vi "initializeGlobals.vi"   [LabVIEW 2015]
uses:
  X:/Lab/Labmembers/Shane Nichols/Labview/InstrumentControl20190423/general_utilities.llb/multiDeviceSynchronization.ctl
  X:/Lab/Labmembers/Shane Nichols/Labview/InstrumentControl20190423/general_utilities.llb/GlobalRefs.vi
  <vilib>/AdaptiveUpright/globalRefs_rigDependent.vi
types:
  T1 = cluster{"galvoX":cluster{"name":string, "physicalChannel":tag}, "galvoY":cluster{"name":string, "physicalChannel":tag}, "mod488":cluster{"name":string, "physicalChannel":tag}, "modTiSaph":cluster{"name":string, "physicalChannel":tag}, "shutter488":cluster{"name":string, "physicalChannel":tag}, "shutterTiSaph":cluster{"name":string, "physicalChannel":tag}, " shutter635":cluster{"name":string, "physicalChannel":tag}, " shutter635-2":cluster{"name":string, "physicalChannel":tag}, "triggerCamera":cluster{"name":string, "physicalChannel":tag}, "triggerBlackfly":cluster{"name":string, "physicalChannel":tag}}
  T2 = cluster{"PMTA":cluster{"name":string, "physicalChannel":tag, "Active?":bool}, "PMTB":cluster{"name":string, "physicalChannel":tag, "Active?":bool}, "cameraExposureOut":cluster{"name":string, "physicalChannel":tag, "Active?":bool}, "galvoPosX":cluster{"name":string, "physicalChannel":tag, "Active?":bool}, "galvoPosY":cluster{"name":string, "physicalChannel":tag, "Active?":bool}, "blackflyCounter":cluster{"name":string, "physicalChannel":tag, "Active?":bool}}
  T3 = typedef "multiDeviceSynchronization.ctl" = cluster{"clockTerminal":tag, "triggerTerminal":tag, "deviceName":string}
  T4 = cluster{"Type":u16, "source":tag, "equivalentChannel":tag}
  T5 = cluster{"name":string, "terminal":tag, "rate":dbl}
  T6 = typedef "LVStringsAndValuesArrayTypeDef_U16.ctl" = cluster{"String":string, "Value":u16}[]
  T7 = cluster{"COM":refnum<visa-resource-name>, "CurrentPosition":u16, "StringsAndValues":T6}[]
  T8 = cluster{"COM":refnum<visa-resource-name>, "CurrentPosition":u16, "StringsAndValues":T6}
  T9 = cluster{"name":string, "terminal":tag, "rate":dbl}[]
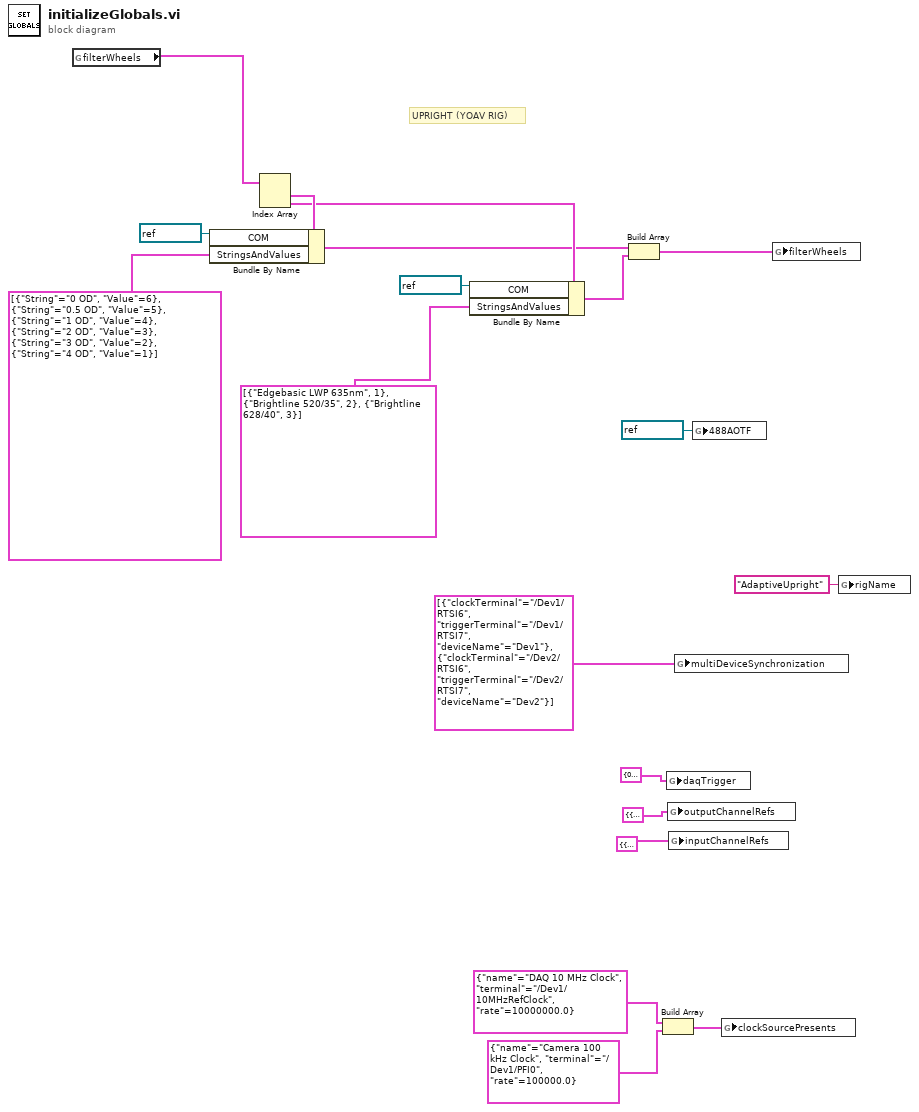
[diagram p0: block diagram]
diagram:
  # "UPRIGHT (YOAV RIG)"
  n1 = global read "GlobalRefs.vi" "filterWheels"() -> (w5:T7)
  n2 = Index Array(array=w5) -> (element #1=w9:T8, element #2=w8:T8)  [unwired: 2 in]
  n3 = Bundle By Name(cluster=w9, "COM"=refnum<visa-resource-name> "COM9", "StringsAndValues"=cluster{"String":string, "Value":u16}[] [{"String"="0 OD", "Value"=6}, {"String"="0.5 OD", "Value"=5}, {"String"="1 OD", "Value"=4}, {"String"="2 OD", "Value"=3}, {"String"="3 OD", "Value"=2}, {"String"="4 OD", "Value"=1}]) -> (w7:T8)
  n4 = Bundle By Name(cluster=w8, "COM"=refnum<visa-resource-name> "COM7", "StringsAndValues"=cluster{string, i32}[] [{"Edgebasic LWP 635nm", 1}, {"Brightline 520/35", 2}, {"Brightline 628/40", 3}]) -> (w6:T8)
  n5 = Build Array(w7, w6) -> (w4:T7)
  n6 = Build Array(T5 {"name"="DAQ 10 MHz Clock", "terminal"="/Dev1/10MHzRefClock", "rate"=10000000.0} ("DAQ 10 MHz Clock"), T5 {"name"="Camera 100 kHz Clock", "terminal"="/Dev1/PFI0", "rate"=100000.0} ("Camera 100 kHz Clock")) -> (w16:T9)
  n7 = global write "globalRefs_rigDependent.vi" "daqTrigger"(T4 {"Type"=0, "source"="/Dev1/PFI3", "equivalentChannel"="Dev1/port1/line3"} ("DAQ_trigger")) -> ()
  n8 = global write "globalRefs_rigDependent.vi" "outputChannelRefs"(T1 {"galvoX"={"name"="galvoX", "physicalChannel"="Dev1/ao0"}, "galvoY"={"name"="galvoY", "physicalChannel"="Dev1/ao1"}, "mod488"={"name"="mod488", "physicalChannel"="Dev1/ao2"}, "modTiSaph"={"name"="modTiSaph", "physicalChannel"="Dev1/ao3"}, "shutter488"={"name"="shutter488", "physicalChannel"="Dev1/port0/line3"}, "shutterTiSaph"={"name"="shutterTiSaph", "physicalChannel"="Dev1/port0/line1"}, " shutter635"={"name"="shutter635", "physicalChannel"="Dev1/port0/line2"}, " shutter635-2"={"name"="shutter635-2", "physicalChannel"="Dev1/port0/line4"}, "triggerCamera"={"name"="triggerCamera", "physicalChannel"="Dev1/port0/line0"}, "triggerBlackfly"={"name"="triggerBlackfly", "physicalChannel"="Dev1/port0/line11"}} ("outputChannelRefs")) -> ()
  n9 = global write "globalRefs_rigDependent.vi" "inputChannelRefs"(T2 {"PMTA"={"name"="PMT1", "physicalChannel"="Dev1/ai0", "Active?"=FALSE}, "PMTB"={"name"="PMT2", "physicalChannel"="Dev1/ai1", "Active?"=FALSE}, "cameraExposureOut"={"name"="cameraExposureOut", "physicalChannel"="Dev1/port0/line6", "Active?"=FALSE}, "galvoPosX"={"name"="galvoPosX", "physicalChannel"="Dev1/ai2", "Active?"=FALSE}, "galvoPosY"={"name"="galvoPosY", "physicalChannel"="Dev1/ai3", "Active?"=FALSE}, "blackflyCounter"={"name"="blackflyCounter", "physicalChannel"="Dev1/port0/line12", "Active?"=FALSE}} ("inputChannelRefs")) -> ()
  n10 = global write "globalRefs_rigDependent.vi" "multiDeviceSynchronization"(T3[] [{"clockTerminal"="/Dev1/RTSI6", "triggerTerminal"="/Dev1/RTSI7", "deviceName"="Dev1"}, {"clockTerminal"="/Dev2/RTSI6", "triggerTerminal"="/Dev2/RTSI7", "deviceName"="Dev2"}] ("multiDeviceSynchronization")) -> ()
  n11 = global write "GlobalRefs.vi" "488AOTF"(refnum<visa-resource-name> "COM6" ("488AOTF")) -> ()
  n12 = global write "globalRefs_rigDependent.vi" "clockSourcePresents"(w16) -> ()
  n13 = global write "GlobalRefs.vi" "filterWheels"(w4) -> ()
  n14 = global write "globalRefs_rigDependent.vi" "rigName"("AdaptiveUpright" ("rigName")) -> ()
